vi "asal sayı bulunca led yakan program .vi"() -> ()   [LabVIEW 2014]
panel:
  out "Boolean":bool
  out "asal 2":dbl[](array[numeric])
  in  "sayı":dbl[](array[numeric])
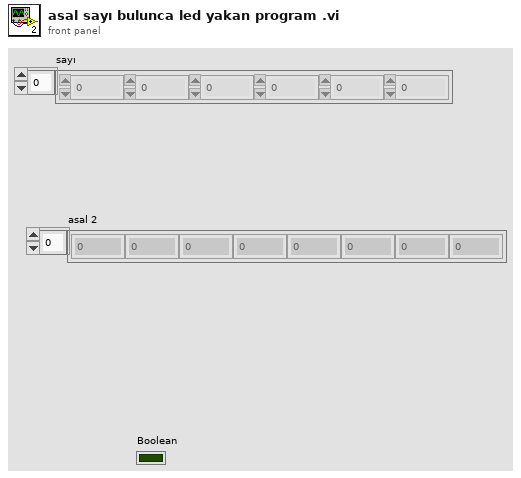
[diagram p1: front panel]
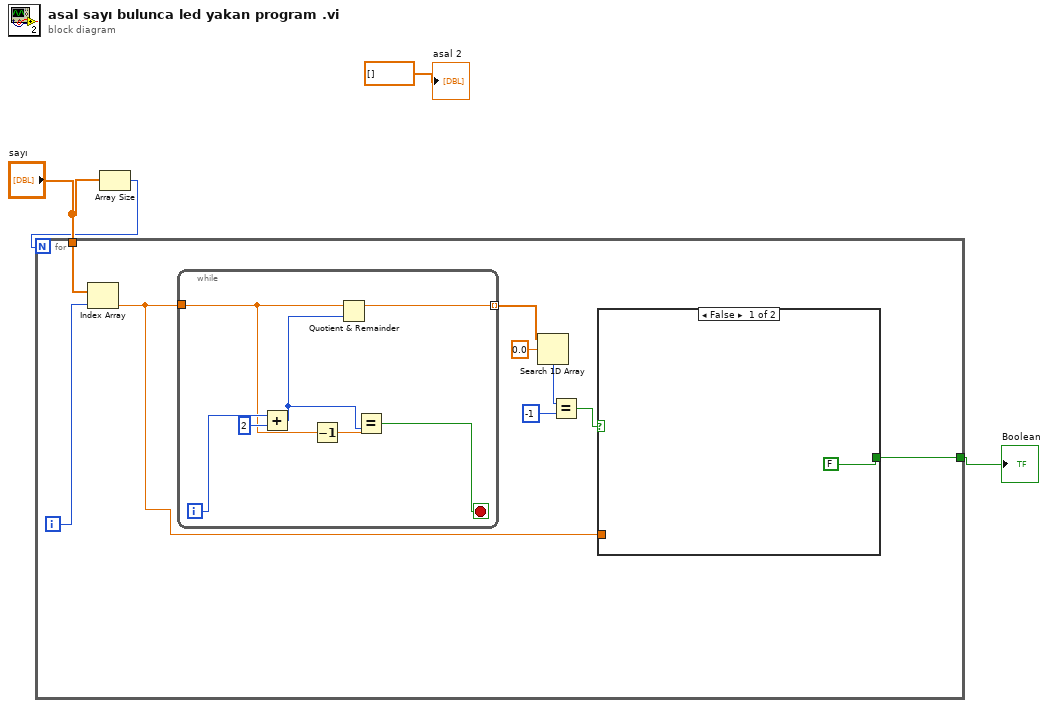
[diagram p0: block diagram]
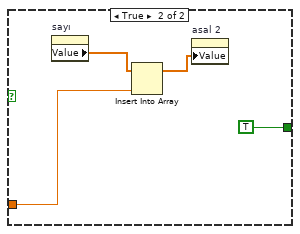
[diagram p2: hidden frame]
diagram:
  n1 = Array Size(array="sayı") -> (size(s)=w2:i32)
  n2 = for {
    N: w2 -> [_]
    tunnel: "sayı" -> [w13]
    tunnel: [w5] -> w1
    i -> [w12]
    n3 = Index Array(array=w13, index=w12) -> (element=w11:dbl)
    n4 = while {
      tunnel: w11 -> [w21]
      tunnel: [w19] -> w10 mode=indexing
      i -> [w24]
      stop <- w20 stop-if-true
      n5 = Add(x=w24, y=2) -> (x+y=w22:i32)
      n6 = Decrement(x=w21) -> (x-1=w25:dbl)
      n7 = Quotient & Remainder(x=w21, y=w22) -> (x-y*floor(x/y)=w19:dbl)  [unwired: 1 out]
      n8 = Equal?(x=w25, y=w22) -> (x = y?=w20:bool)
    }
    n9 = Search 1D Array(1D array=w10, element=0.0) -> (index of element=w8:i32)  [unwired: 1 in]
    n10 = Equal?(x=w8, y=-1) -> (x = y?=w6:bool)
    n11 = case shown="False" w6 {
      tunnel: w11 -> [_ w16]
      tunnel: [FALSE TRUE] -> w5
      frame False {
      }
      frame True {
        n12 = property on="sayı" class="Arr (strict)"() -> ("Value"=w18:dbl[])  [unwired: 2 in, 2 out]
        n13 = Insert Into Array(array=w18, new element=w16) -> (w17:dbl[])  [unwired: 1 in]
        n14 = property on="asal 2" class="Arr (strict)"("Value"=w17) -> ()  [unwired: 2 in, 2 out]
      }
    }
  }
  "Boolean" <- w1
  "asal 2" <- dbl[] [] ("asal 2")
